vi "Comparision Operator.vi"() -> ()   [LabVIEW 2019]
panel:
  out "x <= y?":bool
  out "x >= y?":bool
  out "x != y?":bool
  out "x = y?":bool
  in  "Var 2":u8
  in  "Var1":u8
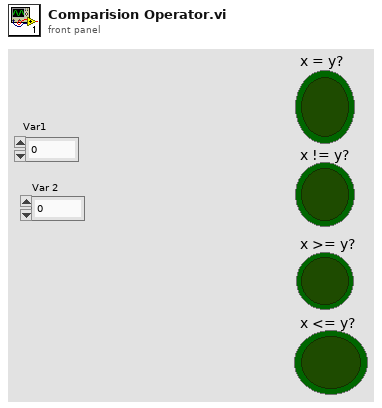
[diagram p1: front panel]
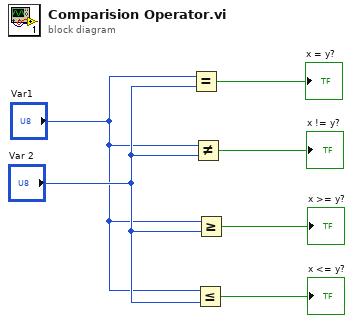
[diagram p0: block diagram]
diagram:
  n1 = Equal?(x="Var1", y="Var 2") -> (x = y?=→"x = y?":bool)
  n2 = Not Equal?(x="Var1", y="Var 2") -> (x != y?=→"x != y?":bool)
  n3 = Less Or Equal?(x="Var1", y="Var 2") -> (x <= y?=→"x <= y?":bool)
  n4 = Greater Or Equal?(x="Var1", y="Var 2") -> (x >= y?=→"x >= y?":bool)
